vi "DeleteNode.vi"(8 "error in (no error)":errorcluster caption="错误输入（无错误）", 10 "Node*":refnum<data-value>, 11 "PanelRootNode 输入":refnum<class "PanelRootNode.lvclass"> caption="DNL_LabVIEW Object in") -> (0 "error out":errorcluster caption="错误输出", 2 "index":i32, 3 "PanelRootNode 输出":refnum<class "PanelRootNode.lvclass"> caption="DNL_LabVIEW Object out")   [LabVIEW 2016, in "PanelRootNode.lvclass"]
uses:
  PanelRootNode.lvclass
  PanelObject/PanelObject.lvclass
  PanelRootNode.lvclass/PanelRootNode.ctl
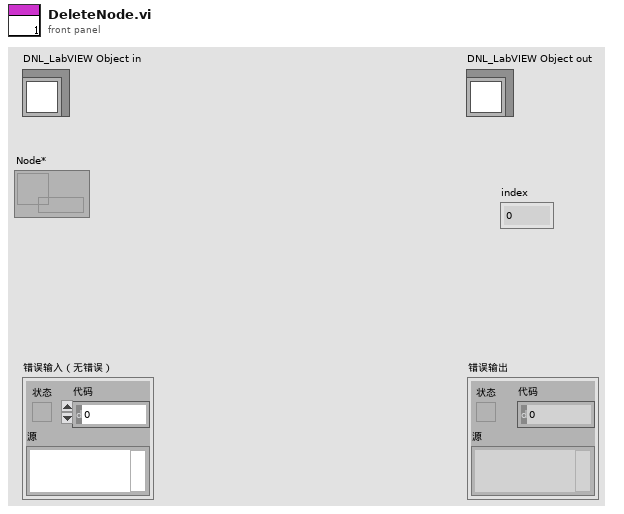
[diagram p1: front panel]
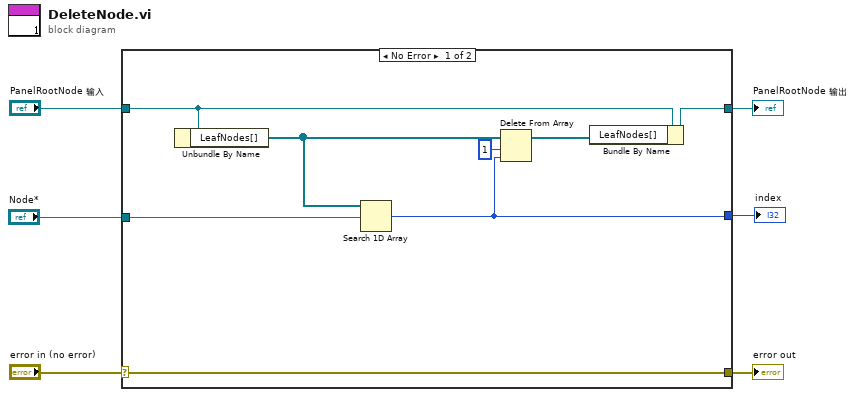
[diagram p0: block diagram]
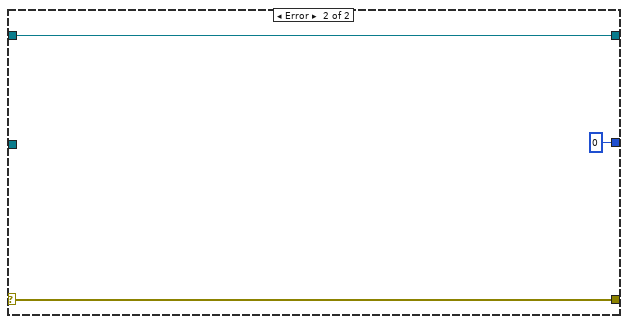
[diagram p2: hidden frame]
diagram:
  n1 = case shown="No Error" "error in (no error)" {
    selector: "error in (no error)" -> [w7 w17]
    tunnel: [w7 w17] -> w5
    tunnel: [w10 w16] -> w3
    tunnel: "PanelRootNode 输入" -> [w12 w16]
    tunnel: "Node*" -> [w8 _]
    tunnel: [w9 0 ("index of element")] -> w1
    frame No Error {
      n2 = Unbundle By Name(w12) -> ("LeafNodes[]"=w14:refnum<data-value>[])
      n3 = Search 1D Array(1D array=w14, element=w8) -> (index of element=w9:i32)  [unwired: 1 in]
      n4 = Delete From Array(array=w14, length=1 ("长度"), index=w9) -> (array with subset deleted=w11:refnum<data-value>[])  [unwired: 1 out]
      n5 = Bundle By Name(cluster=w12, "LeafNodes[]"=w11) -> (w10:refnum<class "PanelRootNode.lvclass">)
    }
    frame Error {
    }
  }
  "error out" <- w5
  "PanelRootNode 输出" <- w3
  "index" <- w1
